vi "Msg.vi"(7 "jettl in":refnum<class "jettl.lvclass">, 11 "Event Last Ack Msg Strategy in":refnum<class "Event Last Ack Msg Strategy.lvclass">) -> (5 "jettl out":refnum<class "jettl.lvclass">)   [LabVIEW 2021, in "jettl.lvlib" / "Event Last Ack.lvlib" / "Event Last Ack Msg Strategy.lvclass"]
uses:
  Event Last Ack Msg Strategy.lvclass
  jettl/jettl.lvclass
  Event Last Ack/Event Last Ack.lvclass
  Event Last Ack Msg Strategy.lvclass/Event Last Ack Msg Strategy.ctl
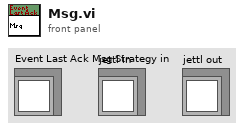
[diagram p1: front panel]
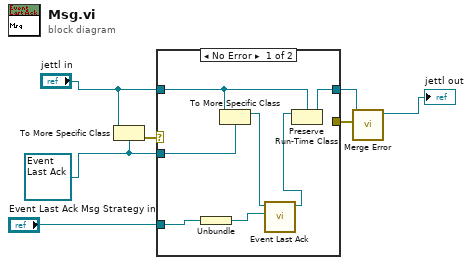
[diagram p0: block diagram]
diagram:
  w2 = refnum<class "Event Last Ack.lvclass"> refnum ("Event Last Ack.lvlib:Event Last Ack.lvclass")
  n1 = To More Specific Class(target class=w2, reference="jettl in") -> (error out=w7:errorcluster)  [unwired: 1 in, 1 out]
  n2 = case shown="No Error" w7 {
    selector: w7 -> [_ w15]
    tunnel: [w12 w16] -> w5
    tunnel: "jettl in" -> [w13 w16]
    tunnel: w2 -> [w14 _]
    tunnel: [_ w15] -> w6
    tunnel: "Event Last Ack Msg Strategy in" -> [w9 _]
    frame No Error {
      n3 = Unbundle(w9) -> (w8:refnum<class "Event jettl.lvclass">)
      n4 = To More Specific Class(target class=w14, reference=w13) -> (specific class reference=w11:refnum<class "Event Last Ack.lvclass">)  [unwired: 1 in, 1 out]
      n5 = call-dynamic "Event Last Ack.vi"("Event jettl"=w8, "Event Last Ack in"=w11) -> ("Event Last Ack out"=w10:refnum<class "Event Last Ack.lvclass">)  [unwired: 9 in]
      n6 = Preserve Run-Time Class(object in=w10, 2:w13) -> (object out=w12:refnum<class "jettl.lvclass">)  [unwired: 1 in, 1 out]
    }
    frame Error {
    }
  }
  n7 = call-dynamic "Merge Error.vi"("Error"=w6, "Merge Error in"=w5) -> ("Merge Error out"=→"jettl out":refnum<class "jettl.lvclass">)  [unwired: 9 in]
